vi "String Create.vi"(8 "error in (no error)":errorcluster, 11 "String value in":string) -> (0 "error out":errorcluster, 3 "String DVR out":refnum<data-value>)   [LabVIEW 2012, in "MDSplus.lvlib"]
uses:
  <vilib>/MDSplus/Library/MDSplus.lvlib
  <vilib>/MDSplus/Classes/Data_Class/Scalar_Class/String_Class/String.lvclass
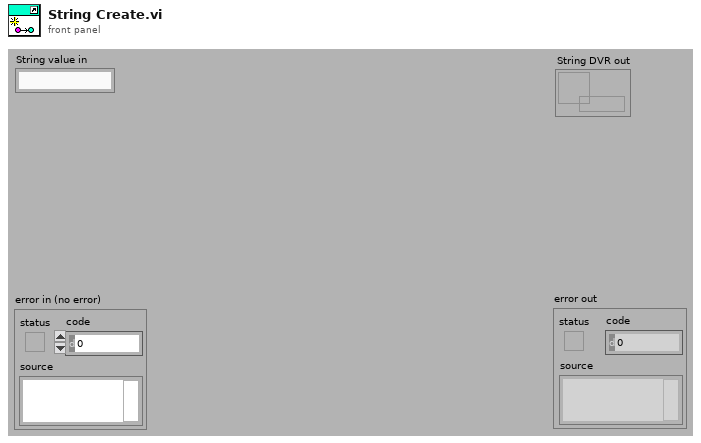
[diagram p1: front panel]
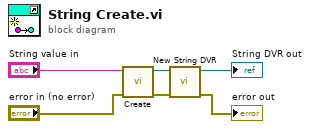
[diagram p0: block diagram]
diagram:
  n1 = call <vilib>:"Create.vi"("error in (no error)"="error in (no error)", "String value in"="String value in") -> ("error out"=w4:errorcluster, "String out"=w5:refnum<class "String.lvclass">)  [unwired: 8 in]
  n2 = call <vilib>:"New String DVR.vi"("error in (no error)"=w4, "String in"=w5) -> ("error out"=→"error out":errorcluster, "String DVR out"=→"String DVR out":refnum<data-value>)  [unwired: 8 in]
